vi "Serial.Find Com Port based on PID and VID.vi"(8 "error in":errorcluster, 10 "PID":string="2500", 11 "VID":string="28DE") -> (0 "error out":errorcluster, 1 "Visa List":string[](array[string]), 2 "Found":bool, 3 "COM Port":string, 5 "Com Ports":string[](array[string]))   [LabVIEW 2018]
uses:
  <vilib>/Instr/_visa.llb/VISA Find Search Mode.ctl
  <vilib>/registry/registry.llb/Registry SAM.ctl
  <vilib>/registry/registry.llb/Read Registry Value Simple STR.vi
panel:
  out "USB Enum Sub Keys":string[](array[string])
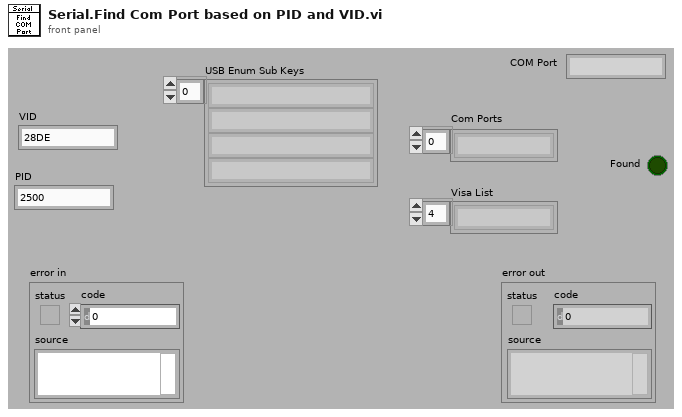
[diagram p1: front panel]
types:
  T1 = typedef "VISA Find Search Mode.ctl" = u32
  T2 = typedef "Registry SAM.ctl" = enum32{"KEY_QUERY_VALUE", "KEY_SET_VALUE", "KEY_CREATE_SUB_KEY", "KEY_ENUMERATE_SUB_KEYS", "KEY_NOTIFY", "KEY_CREATE_LINK", "KEY_READ", "KEY_WRITE", "KEY_ALL_ACCESS", "KEY_READ | KEY_WRITE"}
  T3 = typedef "Registry refnum.ctl" = refnum<k1>
  T4 = cluster{"numSubKeys":i32, "maxSubKeyLen":i32, "maxSubKeyClassLen":i32}
  T5 = cluster{"Root":string, "Enum SubKeys":string[], "SubKeys":string[], "Ports":string[]}
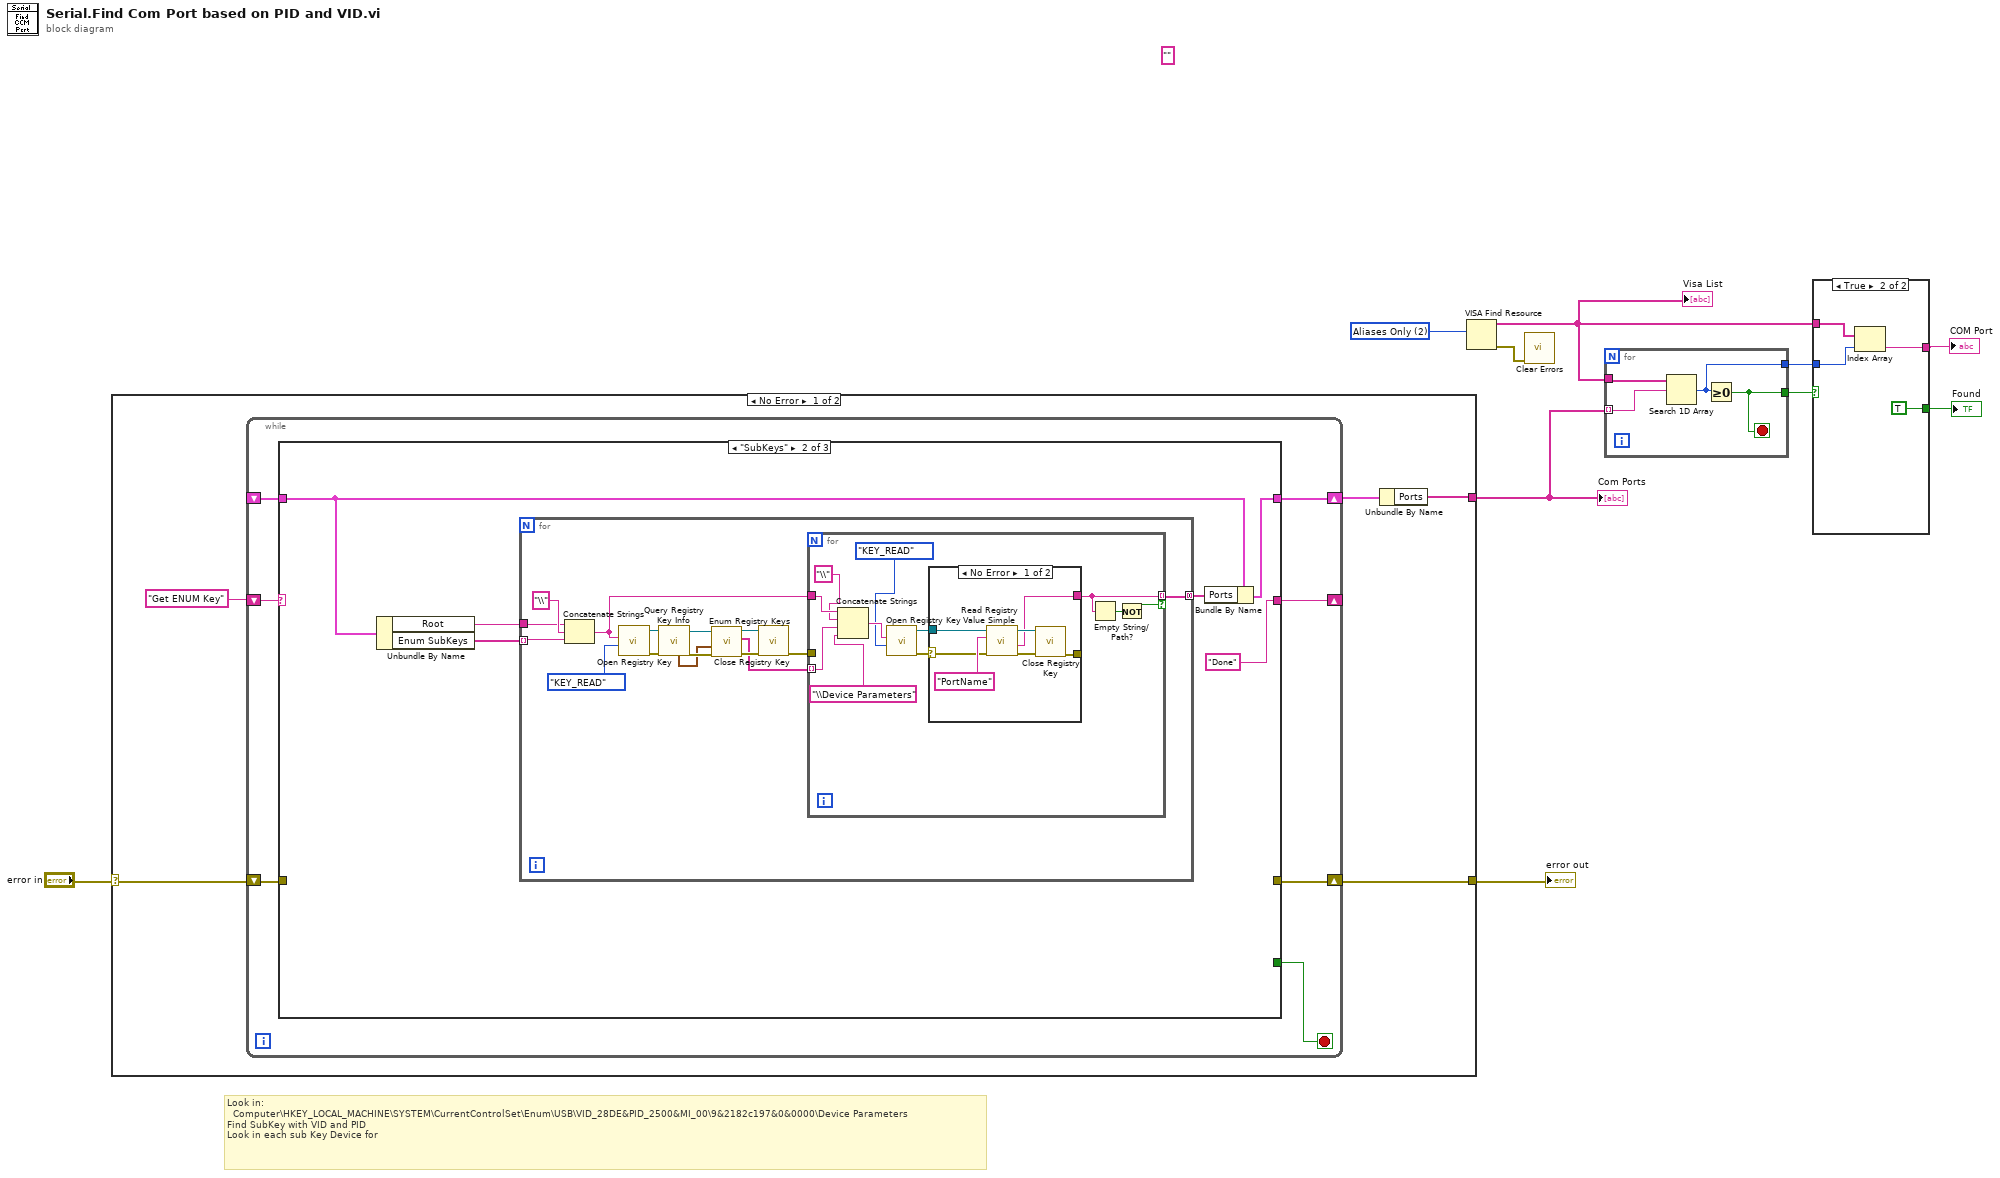
[diagram p0: block diagram]
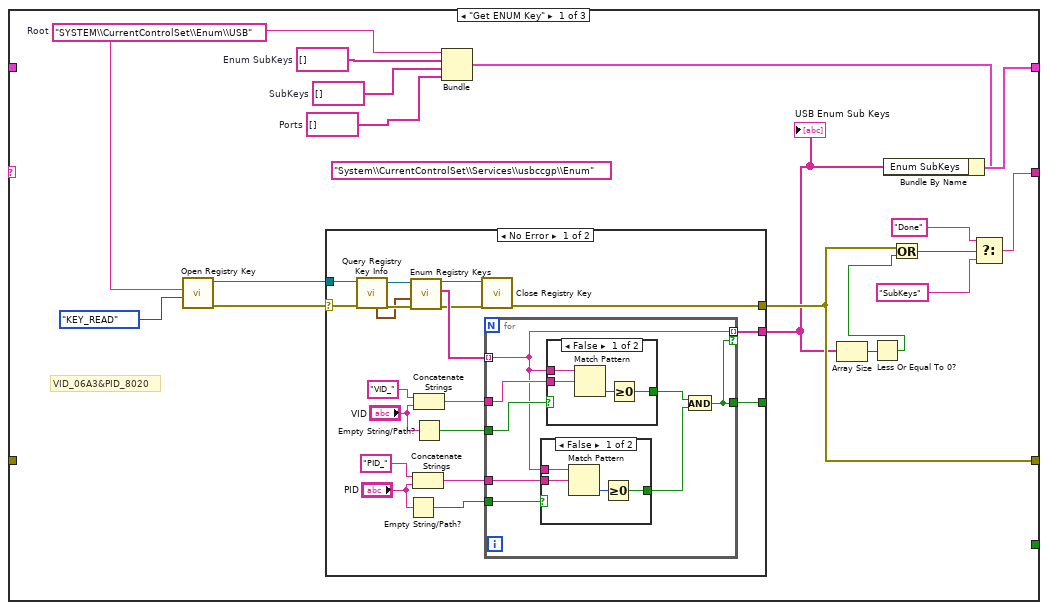
[diagram p3: hidden frame]
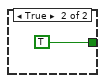
[diagram p4: hidden frame]
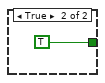
[diagram p5: hidden frame]
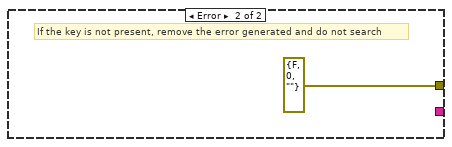
[diagram p6: hidden frame]
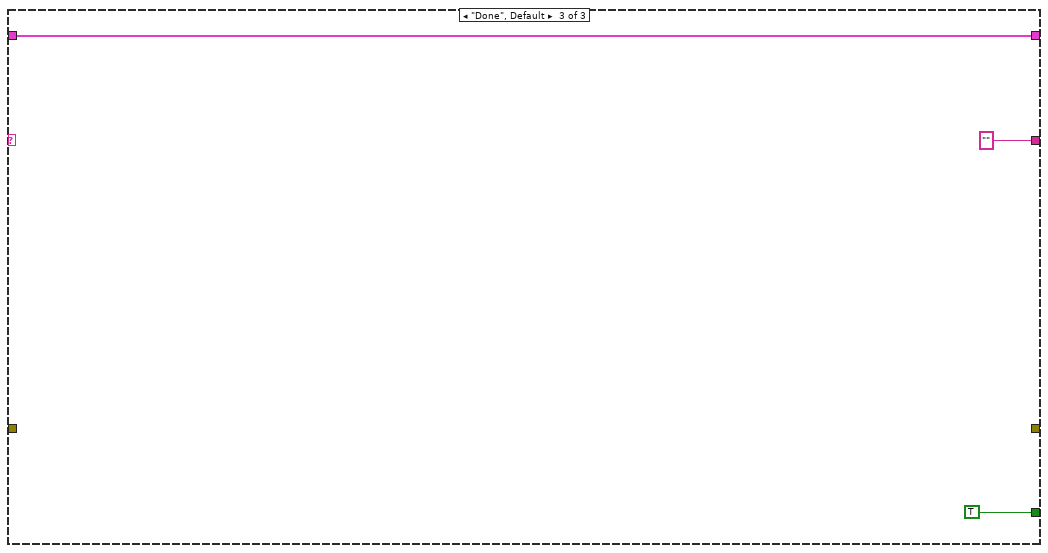
[diagram p8: hidden frame]
diagram:
  w8 = T1 2 items=["Canonical Names Only"=0, "Aliases Only"=2, "Include Matching Aliases"=3, "Include All Aliases"=4] ("Search Mode")
  (unwired) ""
  # "Look in:\n  Computer\\HKEY_LOCAL_MACHINE\\SYSTEM\\CurrentControlSet\\Enum\\USB\\VID_28DE&PID_2500&MI_00\\9&2182c197&0&0000\\Device Parameters\nFind SubKey with VID and PID\nLook in each sub Key Device for"
  n1 = case shown="No Error" "error in" {
    selector: "error in" -> [w11 w120]
    tunnel: [w13 _] -> w7
    tunnel: [w12 w120] -> w10
    frame No Error {
      n2 = while {
        shift-right: [w20] -> w14
        shift-left: _ -> [w21]
        shift-right: [w19] -> w12
        shift-left: w11 -> [w17]
        shift-right: [w18] -> _
        shift-left: "Get ENUM Key" -> [w22]
        stop <- w16 stop-if-true
        n3 = case shown="\"SubKeys\"" w22 {
          tunnel: w21 -> [_ w81 w119]
          tunnel: [w36 w79 w119] -> w20
          tunnel: [w31 _ _] -> w19
          tunnel: [w33 "Done" ""] -> w18
          tunnel: w17 -> [_ _ _]
          tunnel: [_ _ TRUE] -> w16
          frame "Get ENUM Key" {
            w26 = string[] []  # Ports
            w27 = string[] []  # SubKeys
            w29 = string[] []  # Enum SubKeys
            (unwired) "System\\CurrentControlSet\\Services\\usbccgp\\Enum"
            w28 = "SYSTEM\\CurrentControlSet\\Enum\\USB"  # Root
            # "VID_06A3&PID_8020"
            n4 = call <vilib>:"Open Registry Key.vi"("security access mask (KEY_READ | KEY_WRITE)"=Registry_SAM."KEY_READ", "subkey"=w28) -> ("error out"=w38:errorcluster, "refnum out"=w39:T3)  [unwired: 2 in, 6 out]
            n5 = case shown="No Error" w38 {
              selector: w38 -> [w57 _]
              tunnel: w39 -> [w58 _]
              tunnel: [w56 errorcluster {"status"=FALSE, "code"=0, "source"=""} ("error in (no error)")] -> w31
              tunnel: [w47 _] -> _
              tunnel: [w46 _] -> w25
              frame No Error {
                n6 = call <vilib>:"Query Registry Key Info.vi"("error in (no error)"=w57, "refnum"=w58) -> ("error out"=w44:errorcluster, "refnum out"=w45:T3, "subkey info"=w43:T4)  [unwired: 7 out]
                n7 = Empty String/Path?(string/path="PID") -> (empty?=w51:bool)
                n8 = call <vilib>:"Enum Registry Keys.vi"("error in (no error)"=w44, "subkey info"=w43, "refnum"=w45) -> ("error out"=w40:errorcluster, "subkeys"=w42:string[], "refnum out"=w41:T3)  [unwired: 6 in]
                n9 = Concatenate Strings("PID_", "PID") -> (w53:string)
                n10 = Concatenate Strings("VID_", "VID") -> (w50:string)
                n11 = Empty String/Path?(string/path="VID") -> (empty?=w48:bool)
                n12 = call <vilib>:"Close Registry Key.vi"("error in (no error)"=w40, "refnum"=w41) -> ("error out"=w56:errorcluster)  [unwired: 5 out]
                n13 = for {
                  tunnel: w42 -> [w62] mode=indexing
                  tunnel: [w62] -> w46 mode=indexing if=w59
                  tunnel: w50 -> [w64]
                  tunnel: w53 -> [w66]
                  tunnel: w51 -> [w65]
                  tunnel: w48 -> [w63]
                  tunnel: [w59] -> w47
                  n14 = case shown="False" w65 {
                    tunnel: w66 -> [w74 _]
                    tunnel: [w73 TRUE] -> w60
                    tunnel: w62 -> [w72 _]
                    frame False {
                      n15 = Match Pattern(string=w72, regular expression=w74) -> (offset past match=w75:i32)  [unwired: 1 in, 3 out]
                      n16 = Greater Or Equal To 0?(x=w75) -> (x >= 0?=w73:bool)
                    }
                    frame True {
                    }
                  }
                  n17 = case shown="False" w63 {
                    tunnel: w64 -> [w69 _]
                    tunnel: [w68 TRUE] -> w61
                    tunnel: w62 -> [w67 _]
                    frame False {
                      n18 = Match Pattern(string=w67, regular expression=w69) -> (offset past match=w70:i32)  [unwired: 1 in, 3 out]
                      n19 = Greater Or Equal To 0?(x=w70) -> (x >= 0?=w68:bool)
                    }
                    frame True {
                    }
                  }
                  n20 = And(x=w61, y=w60) -> (x .and. y?=w59:bool)
                }
              }
              frame Error {
                # "If the key is not present, remove the error generated and do not search"
              }
            }
            "USB Enum Sub Keys" <- w25
            n21 = Bundle("Root"=w28, "Enum SubKeys"=w29, "SubKeys"=w27, "Ports"=w26) -> (w32:T5)  [unwired: 1 in]
            n22 = Array Size(array=w25) -> (size(s)=w24:i32)
            n23 = Less Or Equal To 0?(x=w24) -> (x <= 0?=w23:bool)
            n24 = Bundle By Name(cluster=w32, "Enum SubKeys"=w25) -> (w36:T5)
            n25 = Or(x=w31, y=w23) -> (x .or. y?=w30:bool)
            n26 = Select(t="Done", s=w30, f="SubKeys") -> (s? t:f=w33:string)
          }
          frame "SubKeys" {
            n27 = Unbundle By Name(w81) -> ("Root"=w83:string, "Enum SubKeys"=w82:string[])
            n28 = for {
              tunnel: w83 -> [w97]
              tunnel: w82 -> [w96] mode=indexing
              tunnel: [w95] -> w80 mode=concatenating
              n29 = Concatenate Strings(w97, "\\", w96) -> (w86:string)
              n30 = call <vilib>:"Open Registry Key.vi"("security access mask (KEY_READ | KEY_WRITE)"=Registry_SAM."KEY_READ", "subkey"=w86) -> ("error out"=w90:errorcluster, "refnum out"=w91:T3)  [unwired: 8 in]
              n31 = call <vilib>:"Query Registry Key Info.vi"("error in (no error)"=w90, "refnum"=w91) -> ("error out"=w93:errorcluster, "refnum out"=w94:T3, "subkey info"=w92:T4)  [unwired: 7 out]
              n32 = call <vilib>:"Enum Registry Keys.vi"("error in (no error)"=w93, "subkey info"=w92, "refnum"=w94) -> ("error out"=w89:errorcluster, "subkeys"=w87:string[], "refnum out"=w88:T3)  [unwired: 6 in]
              n33 = call <vilib>:"Close Registry Key.vi"("error in (no error)"=w89, "refnum"=w88) -> ("error out"=w85:errorcluster)  [unwired: 5 out]
              n34 = for {
                tunnel: [w101] -> w95 mode=indexing if=w100
                tunnel: w87 -> [w107] mode=indexing
                tunnel: w86 -> [w109]
                tunnel: w85 -> [_]
                n35 = Concatenate Strings(w109, "\\", w107, "\\Device Parameters" ("string")) -> (w106:string)
                n36 = call <vilib>:"Open Registry Key.vi"("security access mask (KEY_READ | KEY_WRITE)"=Registry_SAM."KEY_READ", "subkey"=w106) -> ("error out"=w104:errorcluster, "refnum out"=w105:T3)  [unwired: 8 in]
                n37 = case shown="No Error" w104 {
                  selector: w104 -> [w110 _]
                  tunnel: w105 -> [w116 _]
                  tunnel: [w112 _] -> w101
                  tunnel: [w111 _] -> _
                  frame No Error {
                    n38 = call-poly <vilib>:"Read Registry Value Simple.vi"("error in (no error)"=w110, "value"="PortName", "refnum"=w116) -> ("error out"=w113:errorcluster, "String/Binary data"=w112:string, "refnum out"=w114:T3)  [unwired: 3 in, 1 out]
                    n39 = call <vilib>:"Close Registry Key.vi"("error in (no error)"=w113, "refnum"=w114) -> ("error out"=w111:errorcluster)  [unwired: 5 in]
                  }
                  frame Error {
                  }
                }
                n40 = Empty String/Path?(string/path=w101) -> (empty?=w99:bool)
                n41 = Not(x=w99) -> (.not. x?=w100:bool)
              }
            }
            n42 = Bundle By Name(cluster=w81, "Ports"=w80) -> (w79:T5)
          }
          frame "Done", Default {
          }
        }
      }
      n43 = Unbundle By Name(w14) -> ("Ports"=w13:string[])
    }
    frame Error {
    }
  }
  "error out" <- w10
  "Com Ports" <- w7
  n44 = VISA Find Resource(10:w8) -> (0:w1:errorcluster, 3:w6:string[])  [unwired: 2 in, 1 out]
  "Visa List" <- w6
  n45 = call <vilib>:"Clear Errors.vi"("error in (no error)"=w1) -> ()  [unwired: 5 in, 2 out]
  n46 = for {
    tunnel: w6 -> [w124]
    tunnel: w7 -> [w123] mode=indexing
    tunnel: [w122] -> w3
    tunnel: [w121] -> w5
    stop <- w122 stop-if-true
    n47 = Search 1D Array(1D array=w124, element=w123) -> (index of element=w121:i32)  [unwired: 1 in]
    n48 = Greater Or Equal To 0?(x=w121) -> (x >= 0?=w122:bool)
  }
  n49 = case shown="True" w3 {
    tunnel: w6 -> [_ w128]
    tunnel: w5 -> [_ w127]
    tunnel: [_ w126] -> w4
    tunnel: [_ TRUE] -> w2
    frame False {
    }
    frame True {
      n50 = Index Array(array=w128, index=w127) -> (element=w126:string)
    }
  }
  "Found" <- w2
  "COM Port" <- w4
